vi "TestExecuteBasicPolicy_PublishOK.vi"(8 "error in (no error)":errorcluster, 11 "TestCase in":refnum<class "TestSubscriptionPolicy.lvclass">) -> (0 "error out":errorcluster, 3 "TestCase out":refnum<class "TestSubscriptionPolicy.lvclass">)   [LabVIEW 2017, in "TestSubscriptionPolicy.lvclass"]
uses:
  TestSubscriptionPolicy.lvclass
  Transport/QueueTransport/QueueTransport.lvclass/QueueTransport.ctl
  BasicSubscription/BasicSubscription.lvclass/BasicSubscription.ctl
  IMediator/ISubscriptionPolicy/ISubscriptionPolicy.lvclass/ISubscriptionPolicy.ctl
  Transport/QueueTransport/QueueTransport.lvclass
  C:/Git/mva-framework/Framework/IMediator/ITransport/ITransport.lvclass
  BasicSubscription/BasicSubscription.lvclass
  C:/Git/mva-framework/Framework/IMediator/ISubscriptionPolicy/ISubscriptionPolicy.lvclass
  <vilib>/Utility/error.llb/Error Cluster From Error Code.vi
  IMediator/ISubscriptionPolicy/ISubscriptionPolicy.lvclass
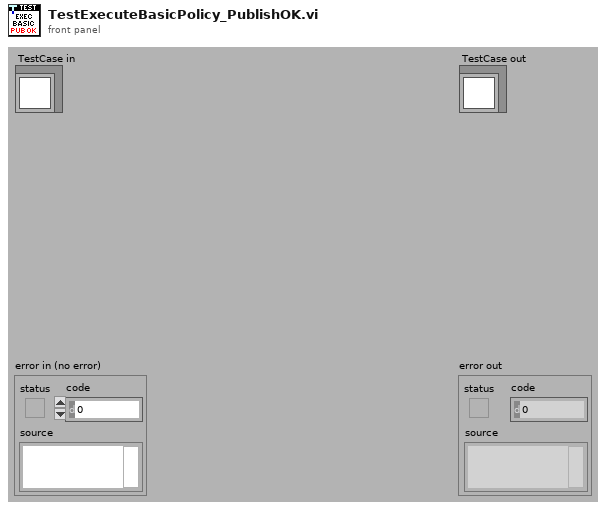
[diagram p1: front panel]
types:
  T1 = typedef "IMediator.lvlib/ISubscriptionPolicy.lvclass/ISubscriptionPolicy Reference.ctl" = refnum<data-value>
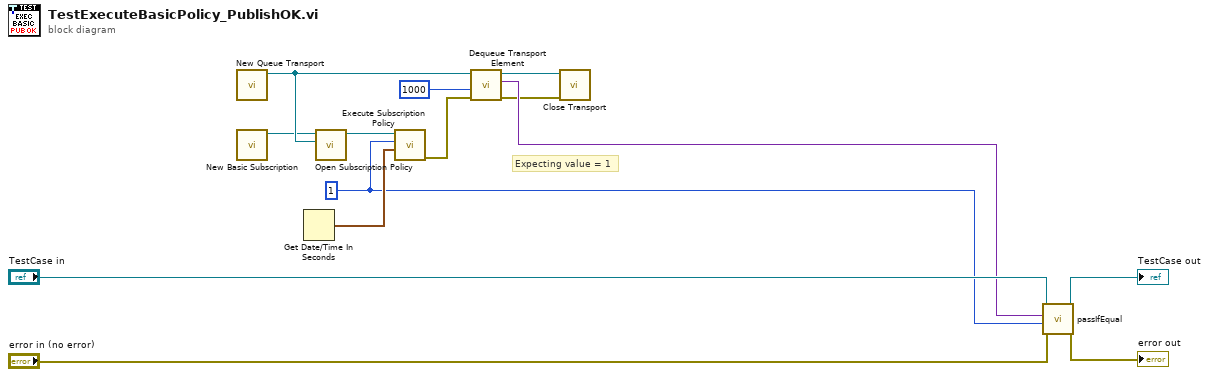
[diagram p0: block diagram]
diagram:
  w2 = 1
  # "Expecting value = 1"
  n1 = call "New Queue Transport.vi"() -> ("QueueTransport"=w9:refnum<class "QueueTransport.lvclass">)  [unwired: 10 in, 1 out]
  n2 = call "New Basic Subscription.vi"() -> ("BasicSubscription Out"=w1:refnum<class "BasicSubscription.lvclass">)  [unwired: 11 in]
  n3 = Get Date/Time In Seconds() -> (seconds since 1Jan1904=w5:timestamp)
  n4 = call "Open Subscription Policy.vi"("Transport"=w9, "SubscriptionPolicy"=w1) -> ("Subscription Policy"=w10:T1)  [unwired: 8 in, 1 out]
  n5 = call "Execute Subscription Policy.vi"("Publish Time"=w5, "New Topic Value"=w2, "Subscription Policy"=w10) -> ("error out (Unsubscribe?)"=w8:errorcluster)  [unwired: 8 in]
  n6 = call "Dequeue Transport Element.vi"("error in (no error)"=w8, "Timeout In ms (-1)"=1000, "QueueTransport in"=w9) -> ("error out"=w3:errorcluster, "Data"=w6:variant, "QueueTransport out"=w4:refnum<class "QueueTransport.lvclass">)  [unwired: 5 in, 1 out]
  n7 = call-dynamic "Close Transport.vi"("error in (no error)"=w3, "QueueTransport in"=w4) -> ()  [unwired: 9 in, 1 out]
  n8 = call-dynamic "passIfEqual.vi"("error in (no error)"="error in (no error)", "y"=w2, "x"=w6, "TestCase in"="TestCase in") -> ("error out"=→"error out":errorcluster, "TestCase out"=→"TestCase out":refnum<class "TestSubscriptionPolicy.lvclass">)  [unwired: 6 in]
